vi "Teleop.vi"(10 "Match Info":T3={"Autonomous Elapsed Seconds"=0.0, "TeleOp Elapsed Seconds"=0.0, "Disabled Elapsed Seconds"=0.0, "Visited Autonomous"=FALSE, "Visited TeleOp"=FALSE, "Visited Disabled"=FALSE, "Autonomous Settings"={"Autonomous Style"=enum."Independent", "VI Refnum"=refnum}}, 11 "Call Context":T4) -> ()   [LabVIEW 2017]
doc: "This VI is called for each TeleOp packet received from the DS where the robot is not disabled. It is often used to read from the joysticks and update I/O or to update setpoints for timed control loops. It should complete and return within 20 milliseconds or it may miss DS packets."
uses:
  <vilib>/Rock Robotics/WPI/DriverStation/WPI_DriverStationDerivedRobotMode.ctl
  <vilib>/Rock Robotics/WPI/DriverStation/WPI_DriverStationMatch Info.ctl
  TypeDefs/dataclusterlocal.ctl
  <vilib>/Rock Robotics/WPI/Solenoid/WPI_SolenoidValue.ctl
  TypeDefs/Localdata.ctl
  TypeDefs/joyaxes.ctl
  <vilib>/Rock Robotics/WPI/ThirdParty/Phoenix-LabVIEW/Motor Controller/Controls/CTRE_Phoenix_MotorControl_ControlMode.ctl
  <vilib>/Rock Robotics/WPI/Utilities/WPI_GetSetVariantRefNum.vi
  <vilib>/Rock Robotics/Network Tables/NT Write Number.vi
  <vilib>/Rock Robotics/WPI/ThirdParty/Phoenix-LabVIEW/Motor Controller/Get/CTRE_Phoenix_MotorController_GetAnalogData.vi
  <vilib>/Rock Robotics/WPI/ThirdParty/Phoenix-LabVIEW/Motor Controller/Get/CTRE_Phoenix_MotorController_GetQuadratureData.vi
  <vilib>/Rock Robotics/WPI/Solenoid/WPI_SolenoidSetEnum.vi
  <vilib>/Rock Robotics/Network Tables/NT Write Numeric Array.vi
  <vilib>/Rock Robotics/Network Tables/NT Read Boolean.vi
  <vilib>/Rock Robotics/Network Tables/NT Read Number.vi
  <vilib>/Rock Robotics/Network Tables/NT Write Boolean Array.vi
panel:
  out "LOOP TIME":dbl
  in  "Teleop local data":T1={"Joy_R_Buttons"=[], "Joy_L_Buttons"=[], "Angular rate"=0.0, "Angle"=0.0, "DriveForwardOutput"=0.0, "TwistOutput"=0.0, "Joy_R_Axes"=[], "Joy_L_Axes"=[], "Fly_L"=0.0, "Fly_R"=0.0, "Pot"=0.0, "LiftOutput"=0.0, "InDrive DeadBand?"=FALSE, "Sol_Clamp"=enum."Reverse", "Sol_RaiseDrop"=enum."Reverse"}
  out "Sample Slider 0":dbl(slide) scale=0.0..5.0
  out "Sample Boolean 1":bool
  out "Sample Boolean 0":bool
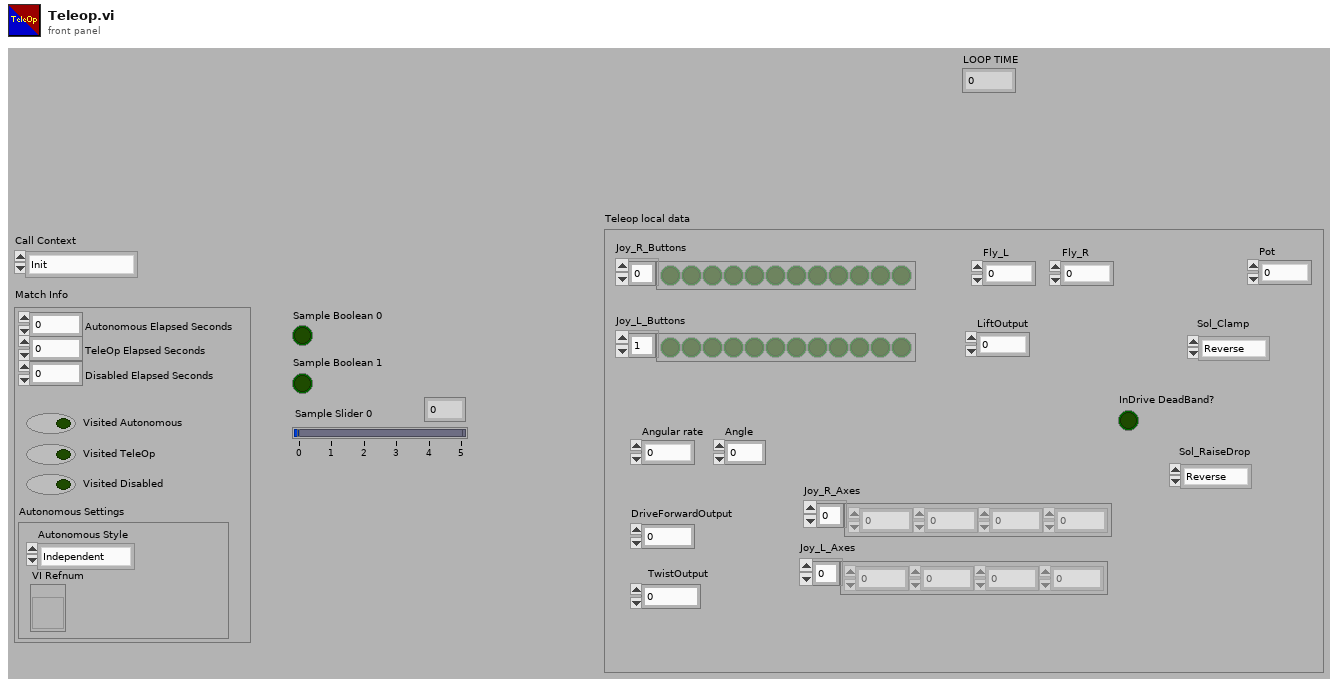
[diagram p1: front panel]
types:
  T1 = typedef "dataclusterlocal.ctl" = cluster{"Joy_R_Buttons":bool[], "Joy_L_Buttons":bool[], "Angular rate":dbl, "Angle":dbl, "DriveForwardOutput":dbl, "TwistOutput":dbl, "Joy_R_Axes":dbl[], "Joy_L_Axes":dbl[], "Fly_L":dbl, "Fly_R":dbl, "Pot":dbl, "LiftOutput":dbl, "InDrive DeadBand?":bool, "Sol_Clamp":T2, "Sol_RaiseDrop":T2}
  T2 = typedef "WPI_SolenoidValue.ctl" = enum16{"Off", "On", "Forward", "Reverse"}
  T3 = typedef "WPI_DriverStationMatch Info.ctl" = cluster{"Autonomous Elapsed Seconds":dbl, "TeleOp Elapsed Seconds":dbl, "Disabled Elapsed Seconds":dbl, "Visited Autonomous":bool, "Visited TeleOp":bool, "Visited Disabled":bool, "Autonomous Settings":cluster{"Autonomous Style":enum16{"Iterative", "Independent"}, "VI Refnum":refnum<vi>}}
  T4 = typedef "WPI_DriverStationDerivedRobotMode.ctl" = enum16{"Init", "Execute", "Stop"}
  T5 = typedef "Localdata.ctl" = enum16{"Start", "i_Joy_R", "i_Joy_L", "i_Gyro", "i_Pot", "i_Encoders", "Calc", "c_DriveForward", "c_DriveTwist", "c_Fly", "c_Lift", "c_Sol", "Outputs", "o_Drive", "o_Fly", "o_Lift", "o_Sol", "End"}
  T6 = typedef "joyaxes.ctl" = enum16{"x axis", "y axis", "twist", "throttle"}
  T7 = typedef "WPI_MotorControlDeviceRef.ctl" = cluster{"DeviceStatus":errorcluster, "Type":T8, "PWM":cluster{"PWM Channel":T9, "DeadBand":T10}, "CAN":cluster{"Device Number":u8, "SetOutput VI Ref":variant, "GetOutput VI Ref":variant, "Enable VI Ref":variant, "Disable VI Ref":variant, "Data":variant}, "Invert":bool, "DIO PWM":cluster{"PWM \"Enable\" Channel":T9, "DIOChannel":T11, "PWM Rate":dbl}}
  T8 = typedef "WPI_MotorControlType.ctl" = enum16{"PWM", "CAN", "DIO PWM"}
  T9 = typedef "FPGA_DIOPWMChannel.ctl" = enum8{"PWM 0", "PWM 1", "PWM 2", "PWM 3", "PWM 4", "PWM 5", "PWM 6", "PWM 7", "PWM 8", "PWM 9", "PWM MXP 0", "PWM MXP 1", "PWM MXP 2", "PWM MXP 3", "PWM MXP 4", "PWM MXP 5", "PWM MXP 6", "PWM MXP 7", "PWM MXP 8", "PWM MXP 9", "Invalid"}
  T10 = typedef "WPI_PWMDeadband.ctl" = cluster{"Name":string, "maxPositivePwm":i32, "minPositivePwm":i32, "centerPwm":i32, "maxNegativePwm":i32, "minNegativePwm":i32, "angularRange":u16}
  T11 = typedef "FPGA_DIOChannel.ctl" = enum8{"DIO 0", "DIO 1", "DIO 2", "DIO 3", "DIO 4", "DIO 5", "DIO 6", "DIO 7", "DIO 8", "DIO 9", "DIO MXP 0", "DIO MXP 1", "DIO MXP 2", "DIO MXP 3", "DIO MXP 4", "DIO MXP 5", "DIO MXP 6", "DIO MXP 7", "DIO MXP 8", "DIO MXP 9", "DIO MXP 10", "DIO MXP 11", "DIO MXP 12", "DIO MXP 13", "DIO MXP 14", "DIO MXP 15", "SPI Port CS1", "SPI Port CS2", "SPI Port CS3", "SPI Port MISO", "SPI Port MOSI", "Invalid"}
  T12 = typedef "WPI_JoystickDevRef.ctl" = cluster{"Device":T13}
  T13 = typedef "WPI_JoystickDeviceEnum.ctl" = enum16{"USB 0", "USB 1", "USB 2", "USB 3", "USB 4", "USB 5"}
  T14 = typedef "WPI_RobotDriveDevRef.ctl" = cluster{"DevStatus":errorcluster, "Motors[]":T7[], "Square Inputs":bool, "Max Output":dbl}
  T15 = typedef "CTRE_Phoenix_MotorControl_ControlMode.ctl" = u16
  T16 = typedef "WPI_SolenoidDevRef.ctl" = cluster{"DevStatus":errorcluster, "Pneumatics Control Module":u8, "Forward Solenoid Channel":T17, "Reverse Solenoid Channel":T17}
  T17 = typedef "WPI_SolenoidChannel.ctl" = enum8{"Solenoid 0", "Solenoid 1", "Solenoid 2", "Solenoid 3", "Solenoid 4", "Solenoid 5", "Solenoid 6", "Solenoid 7", "Invalid"}
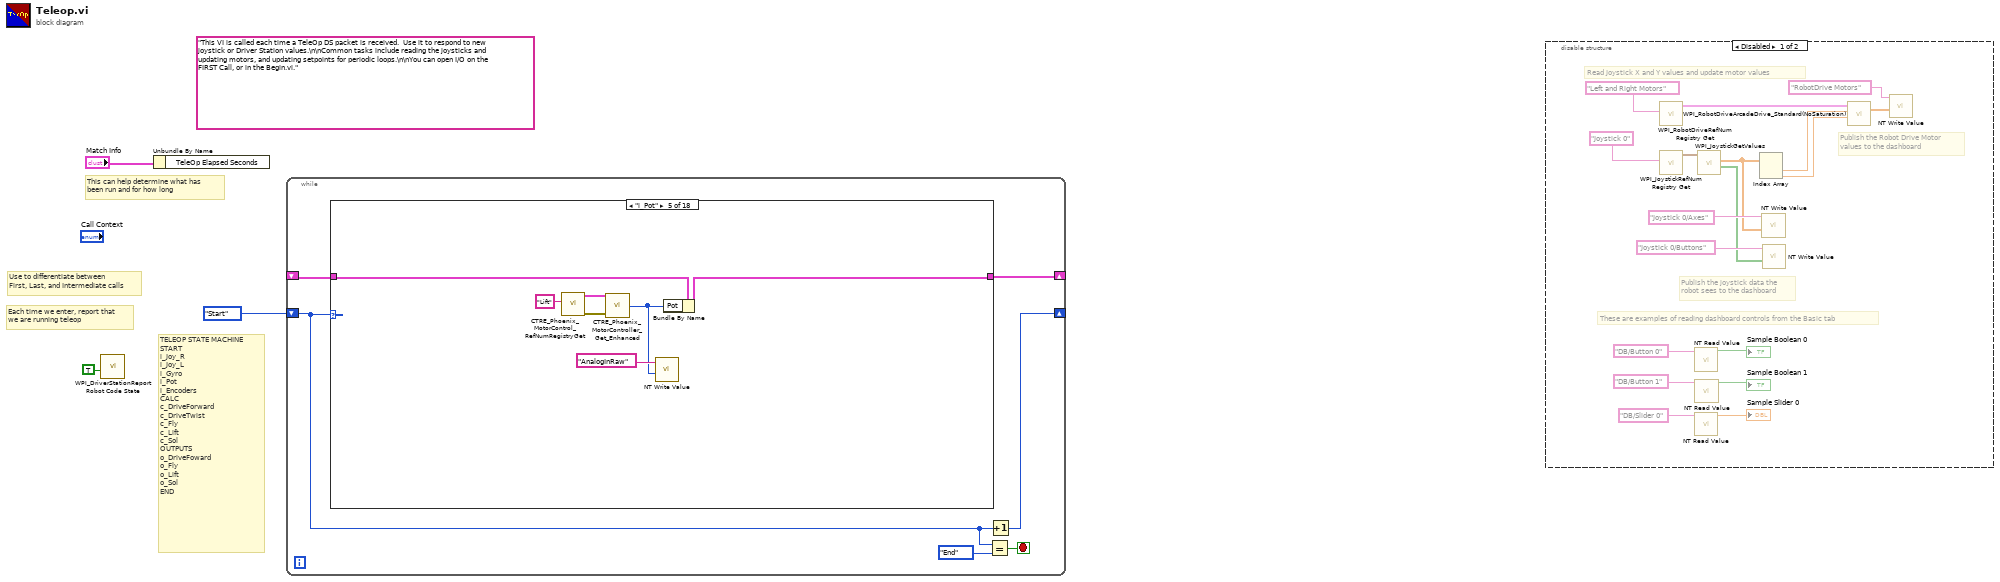
[diagram p0: block diagram]
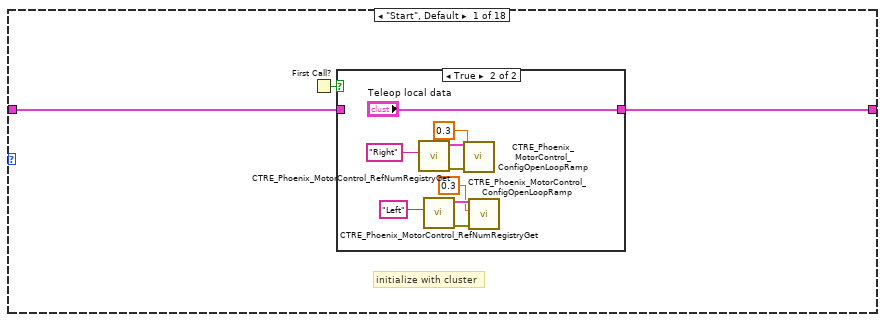
[diagram p2: hidden frame]
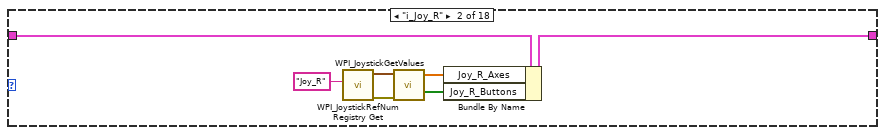
[diagram p4: hidden frame]
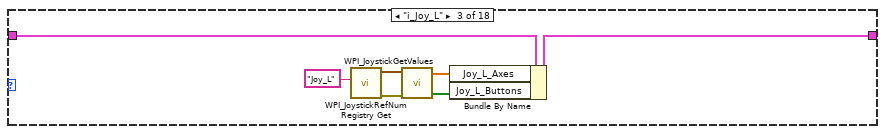
[diagram p5: hidden frame]
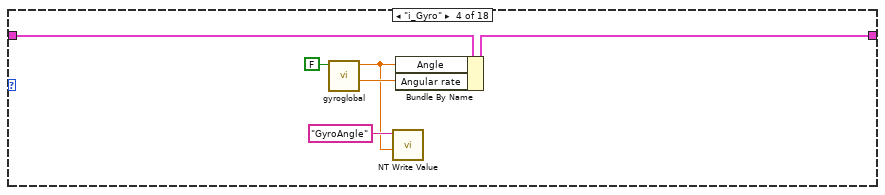
[diagram p6: hidden frame]
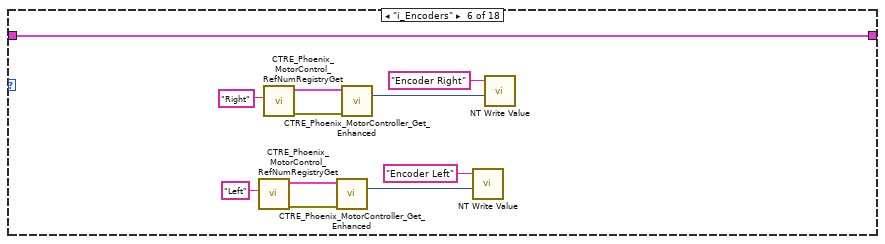
[diagram p7: hidden frame]
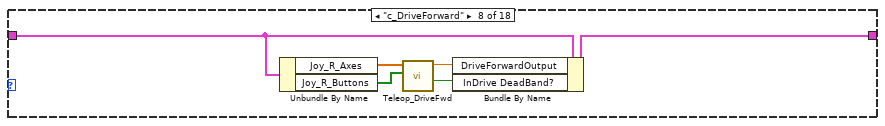
[diagram p9: hidden frame]
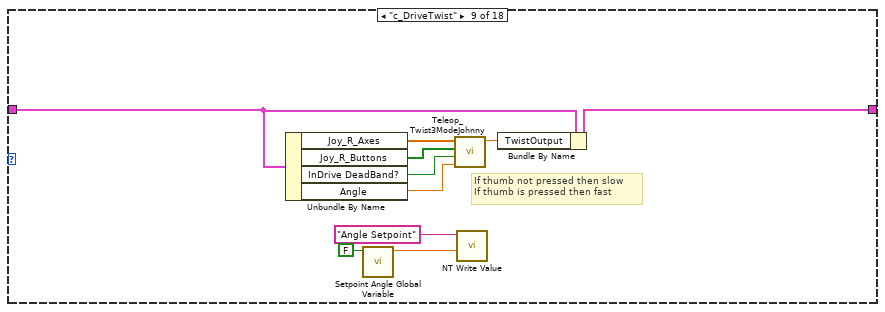
[diagram p10: hidden frame]
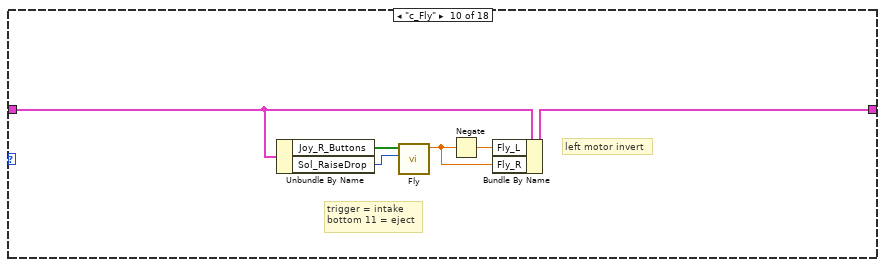
[diagram p11: hidden frame]
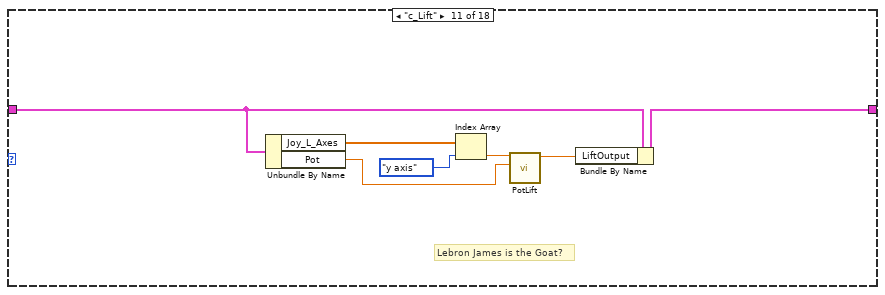
[diagram p12: hidden frame]
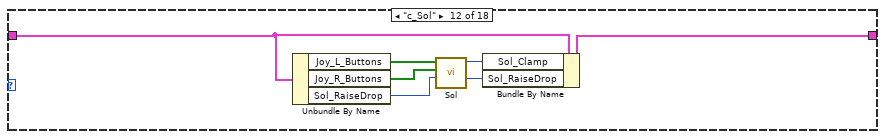
[diagram p13: hidden frame]
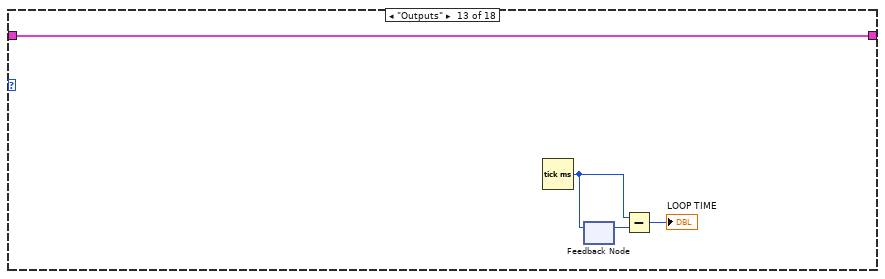
[diagram p14: hidden frame]
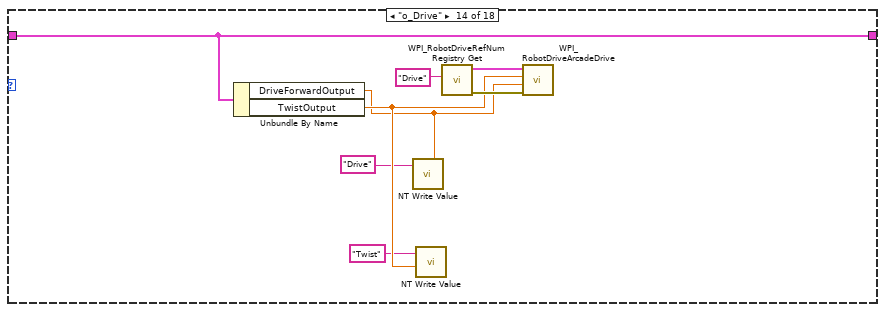
[diagram p15: hidden frame]
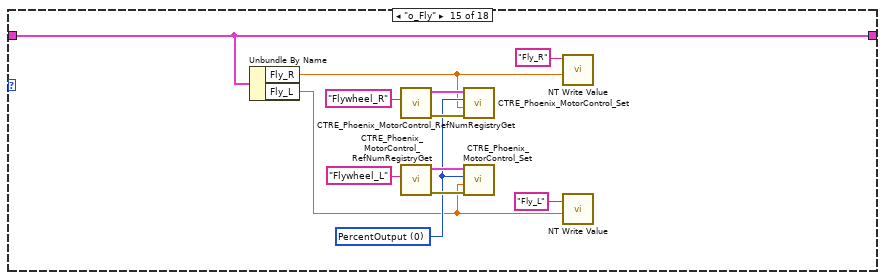
[diagram p16: hidden frame]
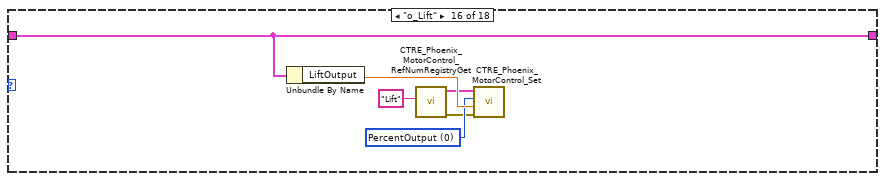
[diagram p17: hidden frame]
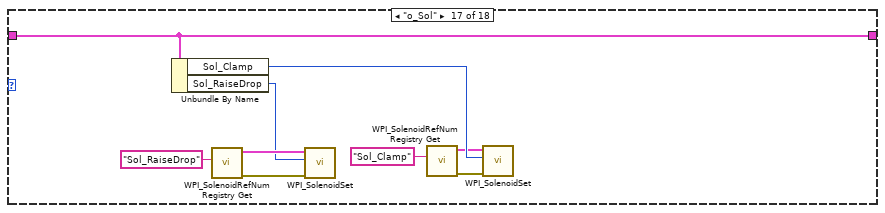
[diagram p18: hidden frame]
diagram:
  (unwired) "This VI is called each time a TeleOp DS packet is received.  Use it to respond to new joystick or Driver Station values.\n\nCommon tasks include reading the joysticks and updating motors, and updating setpoints for periodic loops.\n\nYou can open I/O on the FIRST Call, or in the Begin.vi."
  # "TELEOP STATE MACHINE\nSTART\ni_Joy_R\ni_Joy_L\ni_Gyro\ni_Pot\ni_Encoders\nCALC\nc_DriveForward\nc_DriveTwist\nc_Fly\nc_Lift\nc_Sol\nOUTPUTS\no_DriveFoward\no_Fly\no_Lift\no_Sol\nEND"
  # "Each time we enter, report that\nwe are running teleop"
  # "Use to differentiate between\nFirst, Last, and Intermediate calls"
  # "This can help determine what has\nbeen run and for how long"
  n1 = call <vilib>:"WPI_DriverStationReport Robot Code State.vi"("TeleOp"=TRUE ("Autonomous")) -> ()  [unwired: 10 in, 1 out]
  n2 = Unbundle By Name("Match Info") -> ()  [unwired: 1 out]
  n3 = while {
    shift-right: [w8] -> _
    shift-left: _ -> [w9]
    shift-right: [w5] -> _
    shift-left: Localdata."Start" -> [w4]
    stop <- w6 stop-if-true
    n4 = case shown="\"i_Pot\"" w4 {
      tunnel: w9 -> [w11 w26 w33 w41 w49 w60 w61 w67 w76 w83 w90 w97 w101 w106 w121 w127 w134 w137]
      tunnel: [w10 w25 w32 w40 w48 w60 w61 w66 w77 w82 w88 w96 w101 w106 w121 w127 w134 w137] -> w8
      frame "Start", Default {
        # "initialize with cluster"
        n5 = First Call?() -> (First Call?: T/F=w12:bool)
        n6 = case shown="True" w12 {
          tunnel: [w13 "Teleop local data"] -> w10
          tunnel: w11 -> [w13 _]
          frame False {
          }
          frame True {
            n7 = call <vilib>:"CTRE_Phoenix_MotorControl_RefNumRegistryGet.vi"("refnum name"="Right") -> ("error out"=w21:errorcluster, "PhoenixMotorControlDevRef"=w20:T7)  [unwired: 9 in]
            n8 = call <vilib>:"CTRE_Phoenix_MotorControl_RefNumRegistryGet.vi"("refnum name"="Left") -> ("error out"=w17:errorcluster, "PhoenixMotorControlDevRef"=w16:T7)  [unwired: 9 in]
            n9 = call <vilib>:"CTRE_Phoenix_MotorControl_ConfigOpenLoopRamp.vi"("error in (no error)"=w21, "secondsFromNeutralToFull"=0.3, "PhoenixMotorControlDevRef"=w20) -> ()  [unwired: 7 in, 2 out]
            n10 = call <vilib>:"CTRE_Phoenix_MotorControl_ConfigOpenLoopRamp.vi"("error in (no error)"=w17, "secondsFromNeutralToFull"=0.3, "PhoenixMotorControlDevRef"=w16) -> ()  [unwired: 7 in, 2 out]
          }
        }
      }
      frame "i_Joy_R" {
        n11 = call <vilib>:"WPI_JoystickRefNum Registry Get.vi"("refnum name"="Joy_R") -> ("error out"=w23:errorcluster, "JoystickDevRef"=w28:T12)  [unwired: 9 in]
        n12 = call <vilib>:"WPI_JoystickGetValues.vi"("error in (no error)"=w23, "JoystickDevRef"=w28) -> ("Buttons"=w27:bool[], "Axes"=w24:dbl[])  [unwired: 5 in, 3 out]
        n13 = Bundle By Name(cluster=w26, "Joy_R_Axes"=w24, "Joy_R_Buttons"=w27) -> (w25:T1)
      }
      frame "i_Joy_L" {
        n14 = call <vilib>:"WPI_JoystickRefNum Registry Get.vi"("refnum name"="Joy_L") -> ("error out"=w31:errorcluster, "JoystickDevRef"=w36:T12)  [unwired: 9 in]
        n15 = call <vilib>:"WPI_JoystickGetValues.vi"("error in (no error)"=w31, "JoystickDevRef"=w36) -> ("Buttons"=w30:bool[], "Axes"=w34:dbl[])  [unwired: 5 in, 3 out]
        n16 = Bundle By Name(cluster=w33, "Joy_L_Axes"=w34, "Joy_L_Buttons"=w30) -> (w32:T1)
      }
      frame "i_Gyro" {
        n17 = call "gyroglobal.vi"("Set(T)/Get(F)"=FALSE) -> ("Angular Rate"=w38:dbl, "Angle"=w37:dbl)  [unwired: 9 in]
        n18 = call-poly <vilib>:"NT Write Value.vi"("Numeric"=w37, "Name"="GyroAngle") -> ()  [unwired: 9 in, 1 out]
        n19 = Bundle By Name(cluster=w41, "Angle"=w37, "Angular rate"=w38) -> (w40:T1)
      }
      frame "i_Pot" {
        n20 = call <vilib>:"CTRE_Phoenix_MotorControl_RefNumRegistryGet.vi"("refnum name"="Lift") -> ("error out"=w47:errorcluster, "PhoenixMotorControlDevRef"=w44:T7)  [unwired: 9 in]
        n21 = call-poly <vilib>:"CTRE_Phoenix_MotorController_Get_Enhanced.vi"("PhoenixMotorControlDevRef"=w44, "error in"=w47) -> ("AnalogInRaw"=w43:i32)  [unwired: 9 in, 4 out]
        n22 = call-poly <vilib>:"NT Write Value.vi"("Numeric"=w43, "Name"="AnalogInRaw") -> ()  [unwired: 9 in, 1 out]
        n23 = Bundle By Name(cluster=w49, "Pot"=w43) -> (w48:T1)
      }
      frame "i_Encoders" {
        n24 = call <vilib>:"CTRE_Phoenix_MotorControl_RefNumRegistryGet.vi"("refnum name"="Left") -> ("error out"=w55:errorcluster, "PhoenixMotorControlDevRef"=w52:T7)  [unwired: 9 in]
        n25 = call <vilib>:"CTRE_Phoenix_MotorControl_RefNumRegistryGet.vi"("refnum name"="Right") -> ("error out"=w58:errorcluster, "PhoenixMotorControlDevRef"=w53:T7)  [unwired: 9 in]
        n26 = call-poly <vilib>:"CTRE_Phoenix_MotorController_Get_Enhanced.vi"("PhoenixMotorControlDevRef"=w52, "error in"=w55) -> ("Quadrature Position"=w50:i32)  [unwired: 10 in, 3 out]
        n27 = call-poly <vilib>:"CTRE_Phoenix_MotorController_Get_Enhanced.vi"("PhoenixMotorControlDevRef"=w53, "error in"=w58) -> ("Quadrature Position"=w51:i32)  [unwired: 10 in, 3 out]
        n28 = call-poly <vilib>:"NT Write Value.vi"("Numeric"=w50, "Name"="Encoder Left") -> ()  [unwired: 9 in, 1 out]
        n29 = call-poly <vilib>:"NT Write Value.vi"("Numeric"=w51, "Name"="Encoder Right") -> ()  [unwired: 9 in, 1 out]
      }
      frame "Calc" {
      }
      frame "c_DriveForward" {
        n30 = Unbundle By Name(w67) -> ("Joy_R_Axes"=w64:dbl[], "Joy_R_Buttons"=w63:bool[])
        n31 = call "Teleop_DriveFwd.vi"("Joy_R_Buttons"=w63, "Joy_R_Axes"=w64) -> ("Deadband FWD"=w65:bool, "drive output"=w62:dbl)  [unwired: 8 in]
        n32 = Bundle By Name(cluster=w67, "DriveForwardOutput"=w62, "InDrive DeadBand?"=w65) -> (w66:T1)
      }
      frame "c_DriveTwist" {
        # "If thumb not pressed then slow \nIf thumb is pressed then fast"
        n33 = Unbundle By Name(w76) -> ("Joy_R_Axes"=w71:dbl[], "Joy_R_Buttons"=w70:bool[], "InDrive DeadBand?"=w69:bool, "Angle"=w68:dbl)
        n34 = call "Setpoint Angle Global Variable.vi"("T (Set) F (Get"=FALSE) -> ("Setpoint Angle"=w73:dbl)  [unwired: 10 in]
        n35 = call "Teleop_Twist3ModeJohnny.vi"("Angle"=w68, "In drive deadband?"=w69, "Joy_R_Buttons"=w70, "Joy_R_Axes"=w71) -> ("Twist Output"=w75:dbl)  [unwired: 7 in]
        n36 = call-poly <vilib>:"NT Write Value.vi"("Numeric"=w73, "Name"="Angle Setpoint") -> ()  [unwired: 9 in, 1 out]
        n37 = Bundle By Name(cluster=w76, "TwistOutput"=w75) -> (w77:T1)
      }
      frame "c_Fly" {
        # "trigger = intake\nbottom 11 = eject"
        # "left motor invert"
        n38 = Unbundle By Name(w83) -> ("Joy_R_Buttons"=w80:bool[], "Sol_RaiseDrop"=w78:T2)
        n39 = call "Fly.vi"("Sol_RaiseDrop"=w78, "Joy_R Buttons"=w80) -> ("Flywheel output"=w79:dbl)  [unwired: 9 in]
        n40 = Negate(x=w79) -> (-x=w81:dbl)
        n41 = Bundle By Name(cluster=w83, "Fly_L"=w81, "Fly_R"=w79) -> (w82:T1)
      }
      frame "c_Lift" {
        # "Lebron James is the Goat?"
        n42 = Unbundle By Name(w90) -> ("Joy_L_Axes"=w89:dbl[], "Pot"=w84:dbl)
        n43 = Index Array(array=w89, index=joyaxes."y axis" ("Enum")) -> (element=w86:dbl)
        n44 = call "PotLift.vi"("Pot Position"=w84, "Joystick Y axis"=w86) -> ("Scaled Y"=w85:dbl)  [unwired: 9 in]
        n45 = Bundle By Name(cluster=w90, "LiftOutput"=w85) -> (w88:T1)
      }
      frame "c_Sol" {
        n46 = Unbundle By Name(w97) -> ("Joy_L_Buttons"=w95:bool[], "Joy_R_Buttons"=w91:bool[], "Sol_RaiseDrop"=w92:T2)
        n47 = call "Sol.vi"("Previous Sol_RaiseDrop"=w92, "Joy_L_Buttons"=w91, "Joy_R_Buttons"=w95) -> ("Sol_RaiseDrop"=w93:T2, "Sol_Clamp"=w94:T2)  [unwired: 7 in]
        n48 = Bundle By Name(cluster=w97, "Sol_Clamp"=w94, "Sol_RaiseDrop"=w93) -> (w96:T1)
      }
      frame "Outputs" {
        n49 = Tick Count (ms)() -> (millisecond timer value=w100:u32)
        n50 = feedback-in #1(w100) -> ()
        n51 = feedback #1() -> (w99:u32)  [unwired: 1 in]
        n52 = Subtract(x=w100, y=w99) -> (x-y=→"LOOP TIME":u32)
      }
      frame "o_Drive" {
        n53 = Unbundle By Name(w106) -> ("DriveForwardOutput"=w104:dbl, "TwistOutput"=w105:dbl)
        n54 = call-poly <vilib>:"NT Write Value.vi"("Numeric"=w104, "Name"="Drive") -> ()  [unwired: 9 in, 1 out]
        n55 = call-poly <vilib>:"NT Write Value.vi"("Numeric"=w105, "Name"="Twist") -> ()  [unwired: 9 in, 1 out]
        n56 = call <vilib>:"WPI_RobotDriveRefNum Registry Get.vi"("refnum name"="Drive") -> ("error out"=w107:errorcluster, "RobotDriveDevRef"=w108:T14)  [unwired: 9 in]
        n57 = call-poly <vilib>:"WPI_RobotDriveArcadeDrive.vi"("error in (no error)"=w107, "Y axis value"=w104, "X axis value"=w105, "RobotDriveDevRef"=w108) -> ()  [unwired: 5 in, 3 out]
      }
      frame "o_Fly" {
        w114 = T15 0 items=["PercentOutput"=0, "Position"=1, "Velocity"=2, "Current"=3, "Follower"=5, "MotionProfile"=6, "MotionMagic"=7, "MotionMagicArc"=8, "MotionProfileArc"=10, "Disabled"=15] ("Control Mode")
        n58 = Unbundle By Name(w121) -> ("Fly_R"=w112:dbl, "Fly_L"=w113:dbl)
        n59 = call <vilib>:"CTRE_Phoenix_MotorControl_RefNumRegistryGet.vi"("refnum name"="Flywheel_R") -> ("error out"=w116:errorcluster, "PhoenixMotorControlDevRef"=w120:T7)  [unwired: 9 in]
        n60 = call <vilib>:"CTRE_Phoenix_MotorControl_RefNumRegistryGet.vi"("refnum name"="Flywheel_L") -> ("error out"=w115:errorcluster, "PhoenixMotorControlDevRef"=w119:T7)  [unwired: 9 in]
        n61 = call <vilib>:"CTRE_Phoenix_MotorControl_Set.vi"("error in (no error)"=w116, "Output"=w112, "Control Mode"=w114, "PhoenixMotorControlDevRef"=w120) -> ()  [unwired: 6 in, 2 out]
        n62 = call <vilib>:"CTRE_Phoenix_MotorControl_Set.vi"("error in (no error)"=w115, "Output"=w113, "Control Mode"=w114, "PhoenixMotorControlDevRef"=w119) -> ()  [unwired: 6 in, 2 out]
        n63 = call-poly <vilib>:"NT Write Value.vi"("Numeric"=w112, "Name"="Fly_R") -> ()  [unwired: 9 in, 1 out]
        n64 = call-poly <vilib>:"NT Write Value.vi"("Numeric"=w113, "Name"="Fly_L") -> ()  [unwired: 9 in, 1 out]
      }
      frame "o_Lift" {
        w125 = T15 0 items=["PercentOutput"=0, "Position"=1, "Velocity"=2, "Current"=3, "Follower"=5, "MotionProfile"=6, "MotionMagic"=7, "MotionMagicArc"=8, "MotionProfileArc"=10, "Disabled"=15] ("Control Mode")
        n65 = Unbundle By Name(w127) -> ("LiftOutput"=w126:dbl)
        n66 = call <vilib>:"CTRE_Phoenix_MotorControl_RefNumRegistryGet.vi"("refnum name"="Lift") -> ("error out"=w123:errorcluster, "PhoenixMotorControlDevRef"=w124:T7)  [unwired: 9 in]
        n67 = call <vilib>:"CTRE_Phoenix_MotorControl_Set.vi"("error in (no error)"=w123, "Output"=w126, "Control Mode"=w125, "PhoenixMotorControlDevRef"=w124) -> ()  [unwired: 6 in, 2 out]
      }
      frame "o_Sol" {
        n68 = Unbundle By Name(w134) -> ("Sol_Clamp"=w133:T2, "Sol_RaiseDrop"=w128:T2)
        n69 = call <vilib>:"WPI_SolenoidRefNum Registry Get.vi"("refnum name"="Sol_RaiseDrop") -> ("error out"=w130:errorcluster, "SolenoidDevRef"=w129:T16)  [unwired: 9 in]
        n70 = call-poly <vilib>:"WPI_SolenoidSet.vi"("error in (no error)"=w130, "Value"=w128, "SolenoidDevRef"=w129) -> ()  [unwired: 7 in, 2 out]
        n71 = call <vilib>:"WPI_SolenoidRefNum Registry Get.vi"("refnum name"="Sol_Clamp") -> ("error out"=w135:errorcluster, "SolenoidDevRef"=w132:T16)  [unwired: 9 in]
        n72 = call-poly <vilib>:"WPI_SolenoidSet.vi"("error in (no error)"=w135, "Value"=w133, "SolenoidDevRef"=w132) -> ()  [unwired: 7 in, 2 out]
      }
      frame "End" {
      }
    }
    n73 = Equal?(x=w4, y=Localdata."End") -> (x = y?=w6:bool)
    n74 = Increment(x=w4) -> (x+1=w5:T5)
  }
  n75 = disable-structure shown="Disabled" {
    frame Disabled {
      # "These are examples of reading dashboard controls from the Basic tab"
      # "Publish the Robot Drive Motor\nvalues to the dashboard"
      # "Publish the joystick data the\nrobot sees to the dashboard"
      # "Read Joystick X and Y values and update motor values"
      n76 = call <vilib>:"WPI_RobotDriveRefNum Registry Get.vi"("refnum name"="Left and Right Motors") -> ("RobotDriveDevRef"=w154:T14)  [unwired: 1 in, 9 out]
      n77 = call <vilib>:"WPI_JoystickRefNum Registry Get.vi"("refnum name"="Joystick 0") -> ("JoystickDevRef"=w151:T12)  [unwired: 1 in, 9 out]
      n78 = call-poly <vilib>:"NT Read Value.vi"("Name"="DB/Button 0" ("refnum name")) -> ("Boolean"=→"Sample Boolean 0":bool)  [unwired: 9 in, 1 out]
      n79 = call-poly <vilib>:"NT Read Value.vi"("Name"="DB/Slider 0" ("refnum name")) -> ("Numeric"=→"Sample Slider 0":dbl)  [unwired: 9 in, 1 out]
      n80 = call-poly <vilib>:"NT Read Value.vi"("Name"="DB/Button 1" ("refnum name")) -> ("Boolean"=→"Sample Boolean 1":bool)  [unwired: 9 in, 1 out]
      n81 = call <vilib>:"WPI_JoystickGetValues.vi"("JoystickDevRef"=w151) -> ("Buttons"=w146:bool[], "Axes"=w147:dbl[])  [unwired: 6 in, 3 out]
      n82 = Index Array(array=w147) -> (element #1=w153:dbl, element #2=w150:dbl)  [unwired: 2 in]
      n83 = call-poly <vilib>:"NT Write Value.vi"("Numeric Array"=w147, "Name"="Joystick 0/Axes") -> ()  [unwired: 9 in, 1 out]
      n84 = call-poly <vilib>:"NT Write Value.vi"("Boolean Array"=w146, "Name"="Joystick 0/Buttons") -> ()  [unwired: 9 in, 1 out]
      n85 = call <vilib>:"WPI_RobotDriveArcadeDrive_Standard(NoSaturation).vi"("Y axis value"=w150, "X axis value"=w153, "RobotDriveDevRef"=w154) -> ("Motor Values"=w139:dbl[])  [unwired: 1 in, 7 out]
      n86 = call-poly <vilib>:"NT Write Value.vi"("Numeric Array"=w139, "Name"="RobotDrive Motors") -> ()  [unwired: 9 in, 1 out]
    }
    frame Enabled {
    }
  }
